vi "SMS.vi"(8 "text":string, 11 "phoneNumbers":string[](array[string])) -> ()   [LabVIEW 2014]
uses:
  C:/Users/TGLyt/Documents/GitHub/Daimler/Windows/SubVIs Win/SMSAlerts/SMSAlerts.dll
  Daimler/Windows/SubVIs Win/SMSAlerts/SMSAlerts.dll
panel:
  out "phoneNumbers 2":string[](array[string])
  out "error out":errorcluster
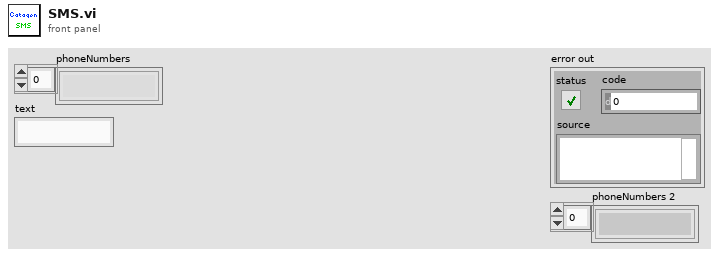
[diagram p1: front panel]
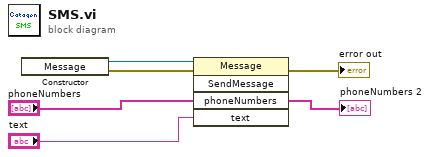
[diagram p0: block diagram]
diagram:
  n1 = constructor class="Message"() -> (reference out=w3:refnum<k24>, error out=w2:errorcluster)  [unwired: 3 in, 1 out]
  n2 = invoke class="Message" method="SendMessage"(reference=w3, error in=w2, "phoneNumbers"="phoneNumbers", "text"="text") -> (error out=→"error out":errorcluster, "phoneNumbers"=→"phoneNumbers 2":string[])  [unwired: 1 in, 3 out]
